vi "CreateTimestampLogFileName.vi"(11 "Time Stamp":timestamp) -> (3 "Timestamp Log File Name":string)   [LabVIEW 2012]
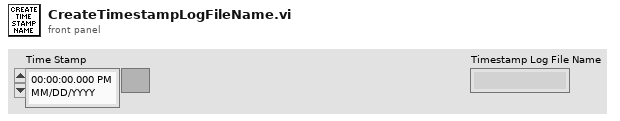
[diagram p1: front panel]
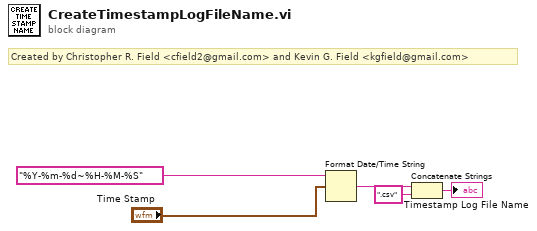
[diagram p0: block diagram]
diagram:
  # "Created by Christopher R. Field <cfield2@gmail.com> and Kevin G. Field <kgfield@gmail.com>"
  n1 = Format Date/Time String(time format string (%c)="%Y-%m-%d~%H-%M-%S", seconds (now)="Time Stamp") -> (date/time string=w4:string)  [unwired: 1 in]
  n2 = Concatenate Strings(w4, ".csv" ("string")) -> (→"Timestamp Log File Name":string)
